vi "Temperature Limit.vi"() -> ()   [LabVIEW 2015]
doc: "This VI simulates the acquisition of temperature, graphs the temperature, and notifies the user if the temperature is over the limit."
panel:
  in  "Start":bool
  in  "Delta t (ms)":i32(slide)=400 scale=50.0..500.0
  in  "Stop":bool
  in  "High Limit":dbl=28.0 format="%.2f"
  out "Temperature":cluster{"Temperature":dbl, "High Limit":dbl}(graph)={"Temperature"=85.88749999999999, "High Limit"=80.0}
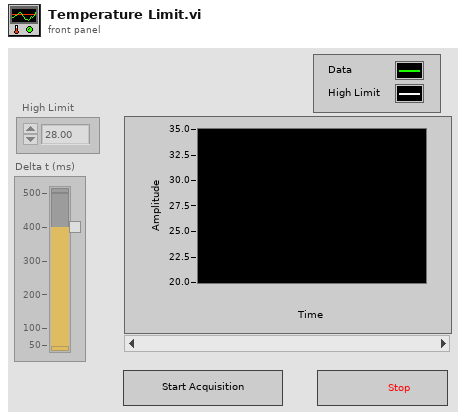
[diagram p1: front panel]
types:
  T1 = enum8{"Enabled", "Disabled", "Disabled and Grayed Out"}
  T2 = cluster{"Temperature Value":dbl, "High Limit":dbl}
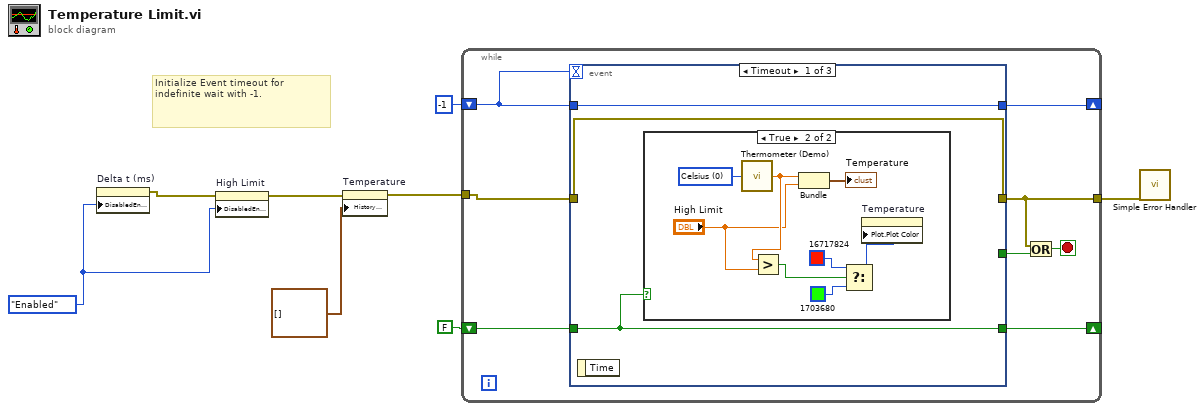
[diagram p0: block diagram]
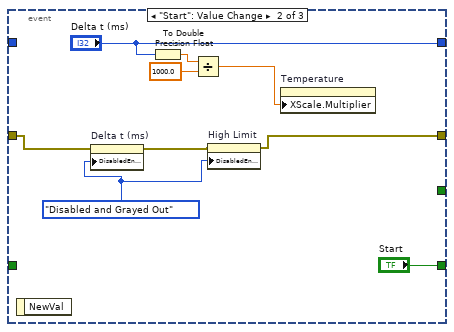
[diagram p3: hidden frame]
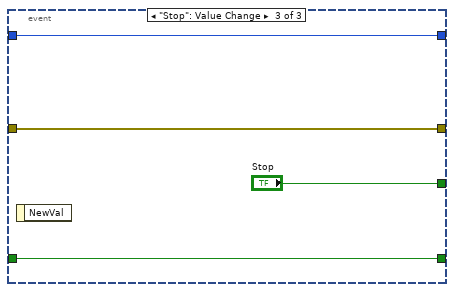
[diagram p4: hidden frame]
diagram:
  w4 = T1."Enabled" ("Disabled")
  # "Initialize Event timeout for indefinite wait with -1."
  n1 = property on="Delta t (ms)" class="Slide (strict)"("DisabledEnum"=w4) -> (error out=w5:errorcluster)  [unwired: 2 in, 1 out]
  n2 = property on="High Limit" class="DigNum (strict)"(error in=w5, "DisabledEnum"=w4) -> (error out=w3:errorcluster)  [unwired: 1 in, 1 out]
  n3 = property on="Temperature" class="WFChart (strict)"(error in=w3, "History Data"=cluster{"Temperature":dbl, "High Limit":dbl}[] []) -> (error out=w2:errorcluster)  [unwired: 1 in, 1 out]
  n4 = while {
    tunnel: [w15] -> w7
    shift-right: [w13] -> _
    shift-left: FALSE ("Start") -> [w12]
    shift-right: [w11] -> _
    shift-left: -1 ("Delta t (ms)") -> [w10]
    tunnel: w2 -> [w9]
    stop <- w16 stop-if-true
    n5 = event shown="[0] Timeout" {
      selector: _ -> [_ _ _]
      dyn-events: _ -> [_ _ _]
      timeout: w10 -> [_ _ _]
      tunnel: [_ _ "Stop"] -> w14
      tunnel: w9 -> [w19 w35 w39]
      tunnel: [w19 w33 w39] -> w15
      tunnel: [w17 "Start" w38] -> w13
      tunnel: w12 -> [w17 _ w38]
      tunnel: [w18 "Delta t (ms)" w37] -> w11
      tunnel: w10 -> [w18 _ w37]
      event Timeout {
        n6 = event-data() -> ()  [unwired: 1 in, 1 out]
        n7 = case shown="True" w17 {
          frame False {
          }
          frame True {
            w26 = u16 0 items=["Celsius", "Fahrenheit"] ("Units (0: Celsius)")
            n8 = call "Thermometer (Demo).vi"("Units (0: Celsius)"=w26) -> ("Temperature Value"=w25:dbl)
            n9 = Greater?(x=w25, y="High Limit") -> (0:w23:bool)
            n10 = Bundle("Temperature Value"=w25, "High Limit"="High Limit") -> (→"Temperature":T2)  [unwired: 1 in]
            n11 = Select(t=u32 16717824, s=w23, f=u32 1703680) -> (s? t:f=w22:u32)
            n12 = property on="Temperature" class="WFChart (strict)"("Plot.Plot Color"=w22) -> ()  [unwired: 2 in, 2 out]
          }
        }
      }
      event "Start": Value Change {
        w32 = T1."Disabled and Grayed Out" ("Disabled")
        n13 = event-data() -> ()  [unwired: 1 in, 1 out]
        n14 = property on="Delta t (ms)" class="Slide (strict)"(error in=w35, "DisabledEnum"=w32) -> (error out=w34:errorcluster)  [unwired: 1 in, 1 out]
        n15 = To Double Precision Float(number="Delta t (ms)") -> (double precision float=w30:dbl)
        n16 = Divide(x=w30, y=1000.0) -> (x/y=w28:dbl)
        n17 = property on="High Limit" class="DigNum (strict)"(error in=w34, "DisabledEnum"=w32) -> (error out=w33:errorcluster)  [unwired: 1 in, 1 out]
        n18 = property on="Temperature" class="WFChart (strict)"("XScale.Multiplier"=w28) -> ()  [unwired: 2 in, 2 out]
      }
      event "Stop": Value Change {
        n19 = event-data() -> ()  [unwired: 1 in, 1 out]
      }
    }
    n20 = Or(x=w15, y=w14) -> (x .or. y?=w16:bool)
  }
  n21 = call <vilib>:"Simple Error Handler.vi"("error in (no error)"=w7) -> ()  [unwired: 4 in, 5 out]
